vi "ArrayToElement.vi"(1 "disabled index (row)":i32, 2 "disabled index (col)":i32, 3 "array":string[][](array[string])) -> (0 "element":string)   [LabVIEW 2011]
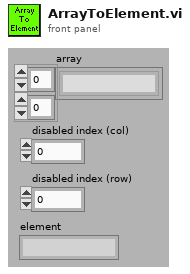
[diagram p1: front panel]
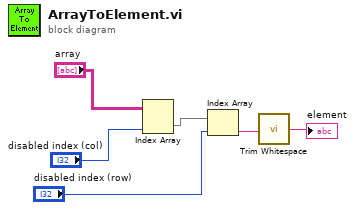
[diagram p0: block diagram]
diagram:
  n1 = Index Array(array="array", index (col)="disabled index (col)") -> (element=w6:string[])  [unwired: 1 in]
  n2 = Index Array(array=w6, index="disabled index (row)") -> (element=w2:string)
  n3 = call <vilib>:"Trim Whitespace.vi"("string"=w2) -> ("trimmed string"=→"element":string)  [unwired: 1 in]
